vi "Remove and Cleanup Device.vi"(8 "error in (no error)":errorcluster, 10 "Device Index":i32, 11 "HAL Editor in":refnum<class "HAL Editor.lvclass">) -> (0 "error out":errorcluster, 3 "HAL Editor out":refnum<class "HAL Editor.lvclass">)   [LabVIEW 2020, in "HAL Config.lvlib" / "HAL Editor.lvclass"]
uses:
  HAL Editor.lvclass
  HAL Editor.lvclass/HAL Editor.ctl
  build/ppl/lv-hal.lvlibp/Device/Device.lvclass
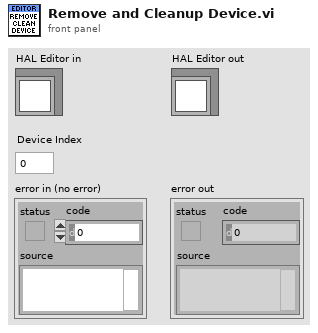
[diagram p1: front panel]
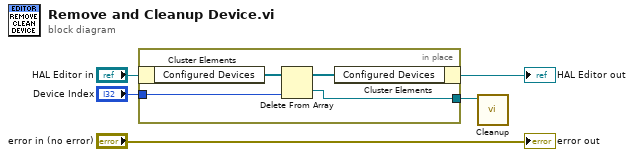
[diagram p0: block diagram]
diagram:
  n1 = in-place {
    in-place-border: "Device Index" -> [w7]
    in-place-border: [w6] -> w1
    n2 = in-place-cluster #1("HAL Editor in") -> ("Configured Devices"=w9:refnum<class "Device.lvclass">[])
    n3 = Delete From Array(array=w9, index=w7) -> (deleted portion=w6:refnum<class "Device.lvclass">, array with subset deleted=w8:refnum<class "Device.lvclass">[])  [unwired: 1 in]
    n4 = in-place-cluster #1("Configured Devices"=w8) -> (→"HAL Editor out":refnum<class "HAL Editor.lvclass">)
  }
  n5 = call "Cleanup.vi"("Device in"=w1) -> ()  [unwired: 10 in, 1 out]
  "error out" <- "error in (no error)"
